vi "Initialize (Simulator).vi"(8 "error in (no error)":errorcluster, 11 "Device ID":T1) -> (0 "error out":errorcluster, 3 "Dynamixel Motor out":refnum<class "Dynamixel Motor.lvclass">)   [LabVIEW 2016, in "Dynamixel Motor Simulator.lvclass"]
doc: "Establishes communication with the sensor. Therefore, call this VI before calling other sensor driver VIs for this sensor. Generally, you need to call the Initialize VI only once at the beginning of an application.\n\n<B>Note:</B>\nYou must call the Start Simulator Service VI on the <B>Robotics>>Simulator</B> palette before calling this VI."
uses:
  <instrlib>/Dynamixel Motor/HAIOL/Simulator/Dynamixel Motor Simulator.lvclass
  <vilib>/robotics/Simulator/Engine/ctl/DeviceID.ctl
  <instrlib>/Dynamixel Motor/HAIOL/Dynamixel Motor.lvclass
  c:/Program Files (x86)/National Instruments/LabVIEW 2016/instr.lib/Dynamixel Motor/HAIOL/Dynamixel Motor.lvclass
  <instrlib>/Dynamixel Motor/HAIOL/Simulator/Dynamixel Motor Simulator.lvclass/Dynamixel Motor Simulator.ctl
  <vilib>/robotics/Simulator/NI_Robotics_Simulator.lvlib
panel:
  # "(c) 2011 National Instruments.  ALL RIGHTS RESERVED."
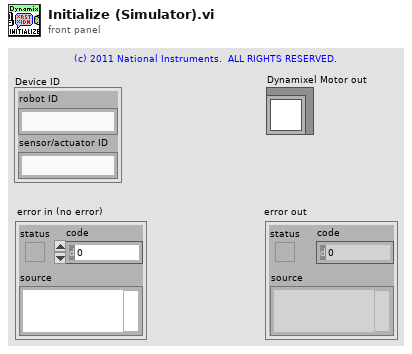
[diagram p1: front panel]
types:
  T1 = typedef "NI_Robotics_Simulator.lvlib/DeviceID.ctl" = cluster{"robot ID":string, "sensor/actuator ID":string}
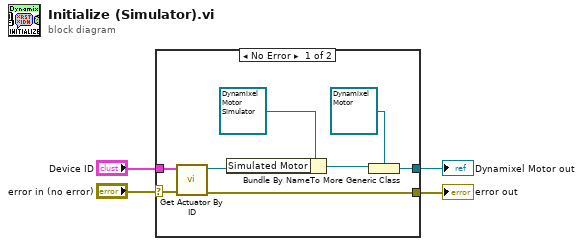
[diagram p0: block diagram]
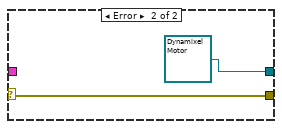
[diagram p2: hidden frame]
diagram:
  n1 = case shown="No Error" "error in (no error)" {
    selector: "error in (no error)" -> [w12 w13]
    tunnel: "Device ID" -> [w11 _]
    tunnel: [w6 refnum<class "Dynamixel Motor.lvclass"> refnum ("Dynamixel Motor.lvclass")] -> w2
    tunnel: [w5 w13] -> w1
    frame No Error {
      n2 = call <vilib>:"Get Actuator By ID.vi"("error in (no error)"=w12, "device ID"=w11) -> ("error out"=w5:errorcluster, "actuator class"=w10:refnum<class "ODESimulator_Motor.lvclass">)  [unwired: 8 in]
      n3 = Bundle By Name(cluster=refnum<class "Dynamixel Motor Simulator.lvclass"> refnum ("Dynamixel Motor Simulator.lvclass"), "Simulated Motor"=w10) -> (w8:refnum<class "Dynamixel Motor Simulator.lvclass">)
      n4 = To More Generic Class(target class=refnum<class "Dynamixel Motor.lvclass"> refnum ("Dynamixel Motor.lvclass"), reference=w8) -> (generic class reference=w6:refnum<class "Dynamixel Motor.lvclass">)
    }
    frame Error {
    }
  }
  "error out" <- w1
  "Dynamixel Motor out" <- w2
